vi "set_temporary_folder_path.vi"(8 "error in (no error)":errorcluster, 10 "Path":path, 11 "Image in":refnum<class "Image.lvclass">) -> (0 "error out":errorcluster, 3 "Image out":refnum<class "Image.lvclass">)   [LabVIEW 2010, in "Image.lvclass"]
uses:
  Image.lvclass
  class_data.vi
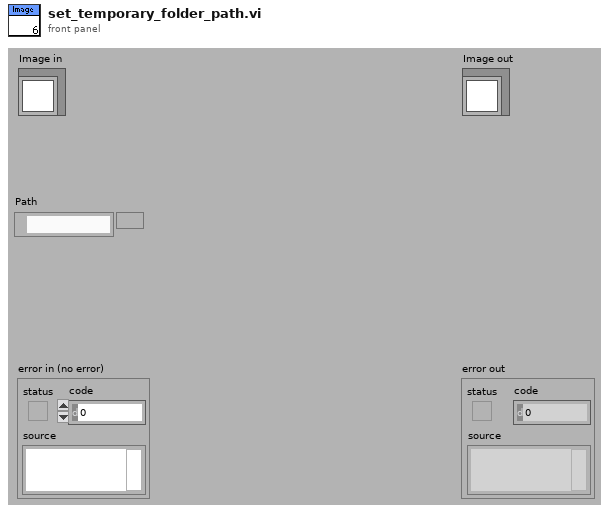
[diagram p1: front panel]
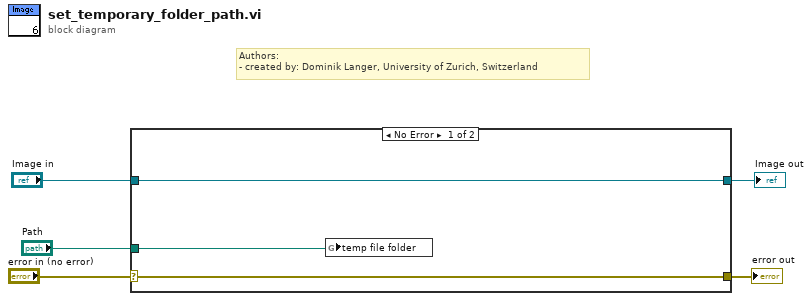
[diagram p0: block diagram]
diagram:
  # "Authors: \n- created by: Dominik Langer, University of Zurich, Switzerland"
  n1 = case shown="No Error" "error in (no error)" {
    selector: "error in (no error)" -> [w7 w10]
    tunnel: [w7 w10] -> w4
    tunnel: [w8 w9] -> w2
    tunnel: "Image in" -> [w8 w9]
    tunnel: "Path" -> [w6 _]
    frame No Error {
      n2 = global write "class_data.vi" "temp file folder"(w6) -> ()
    }
    frame Error {
    }
  }
  "error out" <- w4
  "Image out" <- w2
